vi "fgv_rtcm-msg.vi"(7 "cmd":T1, 11 "rtcm msg":string) -> (3 "rtcm msg out":string)   [LabVIEW 2019]
uses:
  Ctrl/cmd_RW.ctl
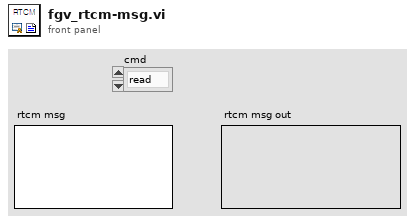
[diagram p1: front panel]
types:
  T1 = typedef "cmd_RW.ctl" = enum16{"read", "write"}
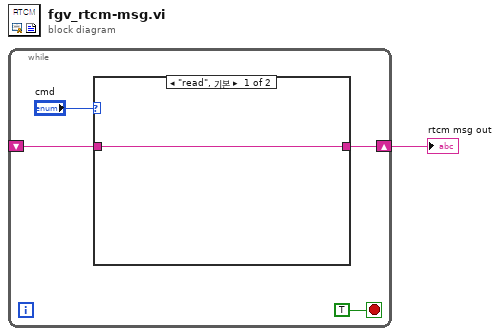
[diagram p0: block diagram]
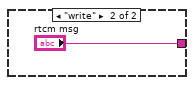
[diagram p2: hidden frame]
diagram:
  n1 = while {
    shift-right: [w3] -> w1
    shift-left: _ -> [w2]
    stop <- TRUE stop-if-true
    n2 = case shown="\"read\", 기본" "cmd" {
      tunnel: [w6 "rtcm msg"] -> w3
      tunnel: w2 -> [w6 _]
      frame "read", Default {
      }
      frame "write" {
      }
    }
  }
  "rtcm msg out" <- w1
